vi "ADD DFS Items One By One.vi"(11 "Tree in":refnum<class "Tree.lvclass">) -> (3 "Tree out":refnum<class "Tree.lvclass">)   [LabVIEW 2022 SP3, in "Tree.lvclass"]
uses:
  Tree.lvclass
  Type Def/Tree Item.ctl
  Tree.lvclass/Tree.ctl
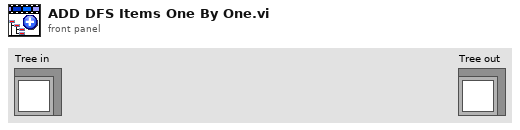
[diagram p1: front panel]
types:
  T1 = typedef "Tree Item.ctl" = cluster{"Parent Tag":string, "Tag":string, "Left Cell":string, "Cells Text":string[], "BFS Index":i32[], "Graph Index":i32, "Item Indent":i32}
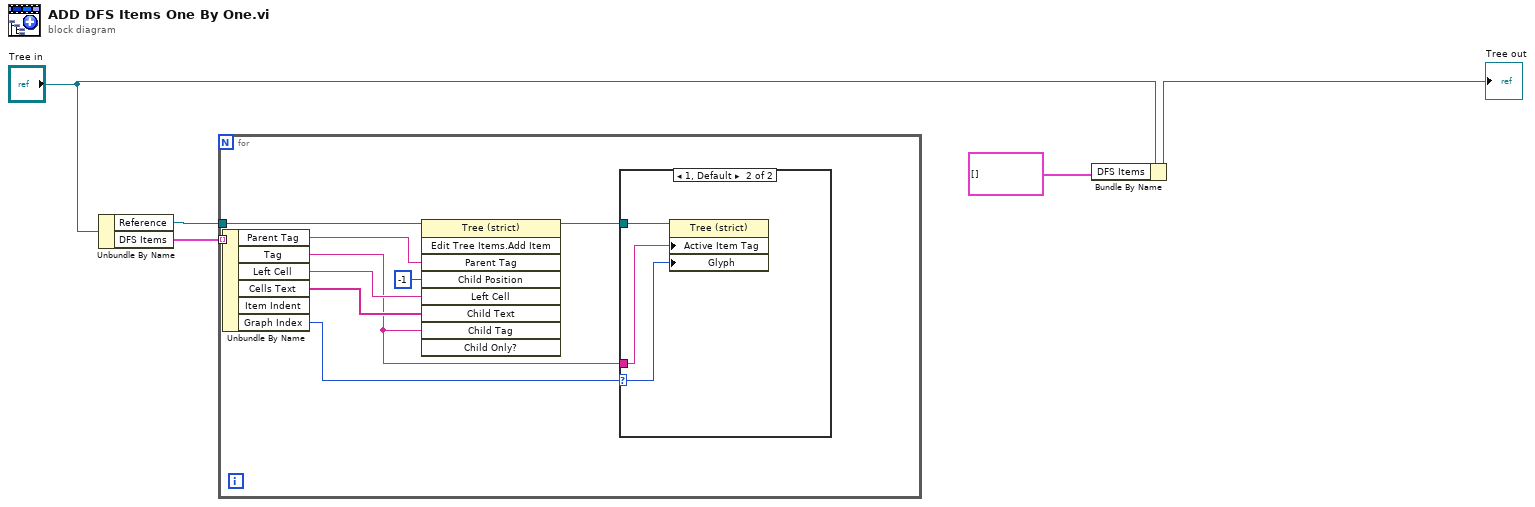
[diagram p0: block diagram]
diagram:
  n1 = Unbundle By Name("Tree in") -> ("Reference"=w4:refnum<vi>, "DFS Items"=w5:T1[])
  n2 = for {
    tunnel: w5 -> [w14] mode=indexing
    tunnel: w4 -> [w13]
    n3 = Unbundle By Name(w14) -> ("Parent Tag"=w12:string, "Tag"=w6:string, "Left Cell"=w10:string, "Cells Text"=w9:string[], "Graph Index"=w8:i32)  [unwired: 1 out]
    n4 = invoke class="Tree (strict)" method="Edit Tree Items.Add Item"(reference=w13, "Parent Tag"=w12, "Child Position"=-1, "Left Cell"=w10, "Child Text"=w9, "Child Tag"=w6) -> (reference out=w7:refnum<vi>)  [unwired: 3 in, 8 out]
    n5 = case shown="1, Default" w8 {
      selector: w8 -> [_ w16]
      tunnel: w7 -> [_ w17]
      tunnel: w6 -> [_ w15]
      frame 0 {
      }
      frame 1, Default {
        n6 = property class="Tree (strict)"(reference=w17, "Active Item Tag"=w15, "Glyph"=w16) -> ()  [unwired: 1 in, 2 out]
      }
    }
  }
  n7 = Bundle By Name(cluster="Tree in", "DFS Items"=T1[] []) -> (→"Tree out":refnum<class "Tree.lvclass">)
